vi "First Step.vi"(8 "error in (no error)":errorcluster, 11 "Continuous.lvclass in":refnum<class "Continuous.lvclass">) -> (0 "error out":errorcluster, 2 "Current Position":dbl, 3 "Continuous.lvclass out":refnum<class "Continuous.lvclass">)   [LabVIEW 2015, in "Continuous.lvclass"]
uses:
  Continuous.lvclass
  Instruments/Magnet/Power Supply/Power Supply.lvclass
  Continuous.lvclass/Continuous.ctl
  Scanner/Scanner.lvclass
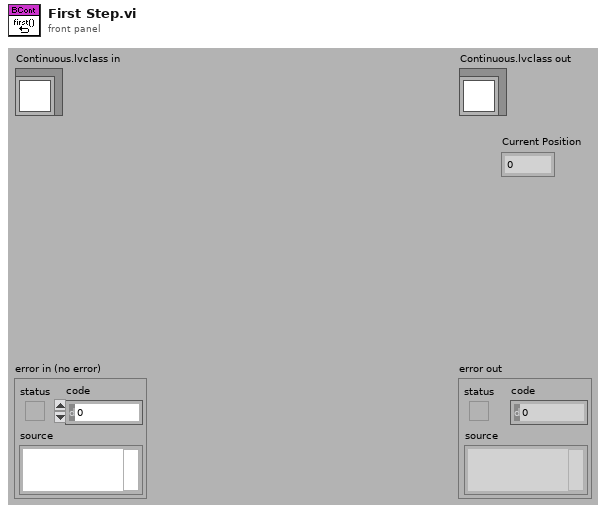
[diagram p1: front panel]
types:
  T1 = typedef "Scanner.lvclass/Range.ctl" = cluster{"xi":dbl, "xf":dbl, "dx":dbl, "Return to...?":bool, "Return to":dbl}
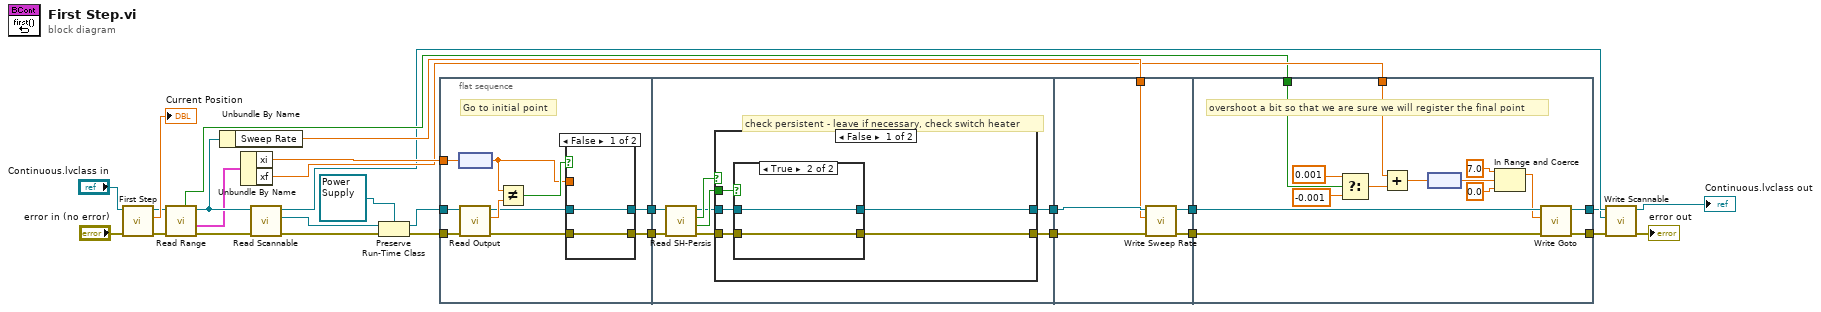
[diagram p0: block diagram]
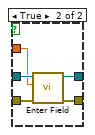
[diagram p2: hidden frame]
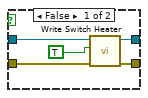
[diagram p3: hidden frame]
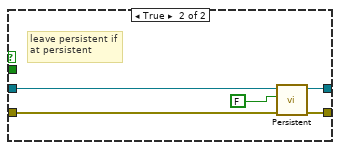
[diagram p4: hidden frame]
diagram:
  n1 = call-parent "First Step.vi"("error in (no error)"="error in (no error)", "Scanner.lvclass in"="Continuous.lvclass in") -> ("error out"=w24:errorcluster, "Current Position"=→"Current Position":dbl, "Scanner.lvclass out"=w25:refnum<class "Continuous.lvclass">)  [unwired: 7 out]
  n2 = call-dynamic "Read Range.vi"("error in (no error)"=w24, "Scanner.lvclass in"=w25) -> ("error out"=w7:errorcluster, "Range"=w1:T1, "Scanner.lvclass out"=w4:refnum<class "Continuous.lvclass">, "Scanning Up?"=w15:bool)  [unwired: 6 out]
  n3 = Unbundle By Name(w4) -> ("Sweep Rate"=w22:dbl[unit])
  n4 = Unbundle By Name(w1) -> ("xi"=w23:dbl, "xf"=w18:dbl)
  n5 = call-dynamic "Read Scannable.vi"("error in (no error)"=w7, "Scanner.lvclass in"=w4) -> ("error out"=w8:errorcluster, "Scannable.lvclass"=w12:refnum<class "Scannable.lvclass">, "Scanner.lvclass out"=w13:refnum<class "Continuous.lvclass">)  [unwired: 7 in]
  n6 = Preserve Run-Time Class(object in=w12, error in=w8, 2:refnum<class "Power Supply.lvclass"> refnum ("Power Supply in")) -> (object out=w10:refnum<class "Power Supply.lvclass">, error out=w9:errorcluster)
  n7 = flat-sequence {
    tunnel: w23 -> [w36]
    tunnel: [w35] -> w21
    tunnel: [w33] -> w16
    tunnel: w10 -> [w30]
    tunnel: w9 -> [w29]
    tunnel: w21 -> [w51]
    tunnel: [w49] -> w20
    tunnel: [w48] -> w17
    tunnel: w16 -> [w46]
    tunnel: w22 -> [w73]
    tunnel: w20 -> [w75]
    tunnel: [w74] -> w19
    tunnel: w17 -> [w72]
    tunnel: [w71] -> w14
    tunnel: w19 -> [w86]
    tunnel: w18 -> [w84]
    tunnel: w15 -> [w83]
    tunnel: w14 -> [w82]
    tunnel: [w81] -> w3
    tunnel: [w80] -> w2
    frame #0 {
      # "Go to initial point"
      n8 = node(w36) -> (w31:dbl[unit])
      n9 = call-dynamic "Read Output.vi"("error in (no error)"=w29, "Power Supply in"=w30) -> ("error out"=w32:errorcluster, "Field"=w38:dbl[unit], "Power Supply out"=w34:refnum<class "Power Supply.lvclass">)  [unwired: 5 in, 2 out]
      n10 = Not Equal?(x=w31, y=w38) -> (x != y?=w37:bool)
      n11 = case shown="False" w37 {
        tunnel: w31 -> [_ w41]
        tunnel: [w40 w45] -> w35
        tunnel: w34 -> [w40 w44]
        tunnel: [w39 w43] -> w33
        tunnel: w32 -> [w39 w42]
        frame False {
        }
        frame True {
          n12 = call-dynamic "Enter Field.vi"("error in (no error)"=w42, "Target field"=w41, "Power Supply in"=w44) -> ("error out"=w43:errorcluster, "Power Supply out"=w45:refnum<class "Power Supply.lvclass">)  [unwired: 7 in]
        }
      }
    }
    frame #1 {
      # "check persistent - leave if necessary, check switch heater"
      n13 = call-dynamic "Read SH-Persis.vi"("error in (no error)"=w46, "Power Supply in"=w51) -> ("error out"=w47:errorcluster, "SHon?"=w53:bool, "pers?"=w52:bool, "Power Supply out"=w50:refnum<class "Power Supply.lvclass">)  [unwired: 4 in, 2 out]
      n14 = case shown="False" w52 {
        tunnel: w53 -> [w58 _]
        tunnel: w50 -> [w56 w69]
        tunnel: [w55 w68] -> w49
        tunnel: [w54 w67] -> w48
        tunnel: w47 -> [w57 w66]
        frame False {
          n15 = case shown="True" w58 {
            tunnel: w57 -> [w63 w65]
            tunnel: w56 -> [w62 w64]
            tunnel: [w61 w64] -> w55
            tunnel: [w60 w65] -> w54
            frame False {
              n16 = call-dynamic "Write Switch Heater.vi"("error in (no error)"=w63, "Turn SH On?"=TRUE, "Power Supply in"=w62) -> ("error out"=w60:errorcluster, "Power Supply out"=w61:refnum<class "Power Supply.lvclass">)  [unwired: 7 in]
            }
            frame True {
            }
          }
        }
        frame True {
          # "leave persistent if\nat persistent"
          n17 = call-dynamic "Persistent.vi"("error in (no error)"=w66, "Go to persistent mode?"=FALSE, "Power Supply in"=w69) -> ("error out"=w67:errorcluster, "Power Supply out"=w68:refnum<class "Power Supply.lvclass">)  [unwired: 7 in]
        }
      }
    }
    frame #2 {
      n18 = call-dynamic "Write Sweep Rate.vi"("error in (no error)"=w72, "rate"=w73, "Power Supply in"=w75) -> ("error out"=w71:errorcluster, "Power Supply out"=w74:refnum<class "Power Supply.lvclass">)  [unwired: 7 in]
    }
    frame #3 {
      # "overshoot a bit so that we are sure we will register the final point"
      n19 = Select(t=0.001, s=w83, f=-0.001) -> (s? t:f=w89:dbl)
      n20 = Add(x=w84, y=w89) -> (x+y=w85:dbl)
      n21 = node(w85) -> (w77:dbl[unit])
      n22 = In Range and Coerce(upper limit=dbl[unit] 7.0, x=w77, lower limit=dbl[unit] 0.0) -> (coerced(x)=w76:dbl[unit])  [unwired: 1 out]
      n23 = call-dynamic "Write Goto.vi"("error in (no error)"=w82, "Target"=w76, "Power Supply in"=w86) -> ("error out"=w80:errorcluster, "Power Supply out"=w81:refnum<class "Power Supply.lvclass">)  [unwired: 7 in]
    }
  }
  n24 = call-dynamic "Write Scannable.vi"("error in (no error)"=w2, "Scannable.lvclass"=w3, "Scanner.lvclass in"=w13) -> ("error out"=→"error out":errorcluster, "Scanner.lvclass out"=→"Continuous.lvclass out":refnum<class "Continuous.lvclass">)  [unwired: 7 in]
